vi "Log Current Register Values.vi"(7 "Unit ID (A)":string="A", 8 "error in":errorcluster, 10 "Use VI path? (T)":bool=TRUE, 11 "VISA Session In":refnum<visa-resource-name>="Alicat") -> (0 "error out":errorcluster, 3 "VISA Session Out":refnum<visa-resource-name>)   [LabVIEW 2014]
doc: "Reads off the value in each configuration/diagnostic register, and stores the values in a text file. Alicat saves a register log of each device before it leaves our facility; please contact us at (520) 290-6060 or by email at info@alicat.com if you are in need of this log file."
uses:
  <vilib>/Utility/file.llb/Write To Spreadsheet File (string).vi
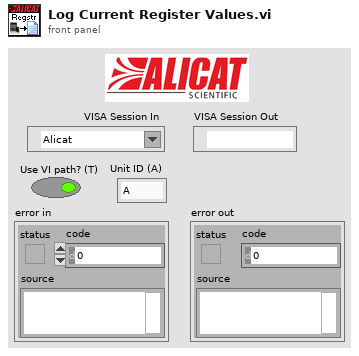
[diagram p1: front panel]
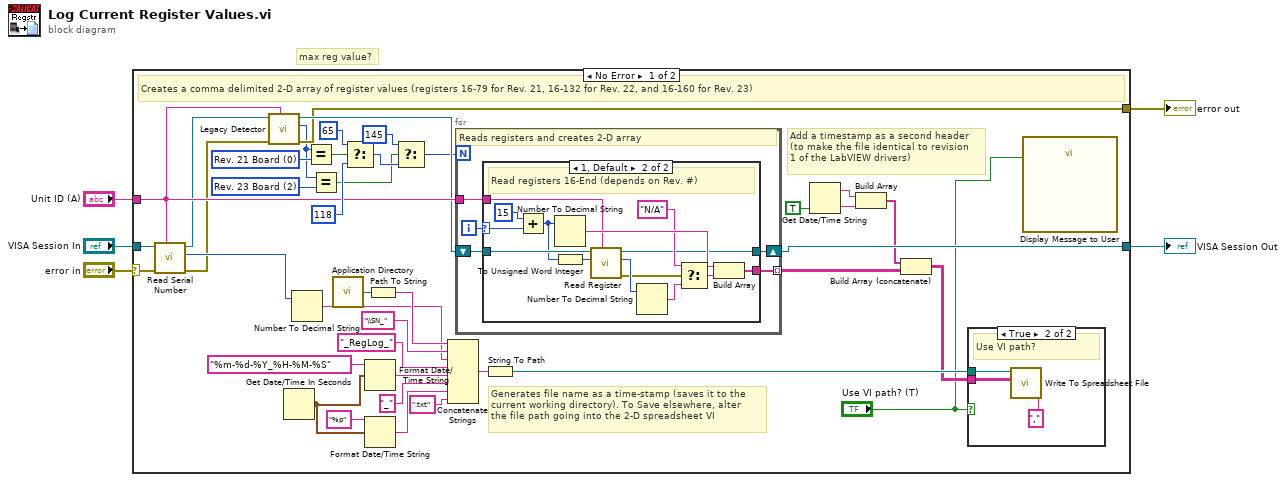
[diagram p0: block diagram]
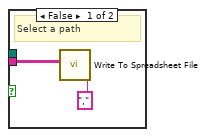
[diagram p2: hidden frame]
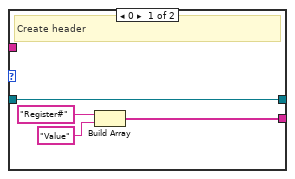
[diagram p3: hidden frame]
diagram:
  # "max reg value?"
  n1 = case shown="No Error" "error in" {
    selector: "error in" -> [w40 w75]
    tunnel: "VISA Session In" -> [w44 w74]
    tunnel: "Unit ID (A)" -> [w24 _]
    tunnel: [w43 w74] -> w3
    tunnel: [w20 w75] -> w2
    frame No Error {
      w9 = u8 2 items=["Rev. 21 Board", "Rev. 22 Board", "Rev. 23 Board"] ("Legacy Status")
      w45 = u8 0 items=["Rev. 21 Board", "Rev. 22 Board", "Rev. 23 Board"] ("Legacy Status")
      # "Add a timestamp as a second header\n(to make the file identical to revision\n1 of the LabVIEW drivers)"
      # "Generates file name as a time-stamp (saves it to the \ncurrent working directory). To Save elsewhere, alter\nthe file path going into the 2-D spreadsheet VI"
      # "Creates a comma delimited 2-D array of register values (registers 16-79 for Rev. 21, 16-132 for Rev. 22, and 16-160 for Rev. 23)"
      n2 = call "Read Serial Number.vi"("Unit ID (A)"=w24, "error in"=w40, "VISA Session In"=w44) -> ("error out"=w21:errorcluster, "Serial Number"=w26:i32, "VISA Session Out"=w23:refnum<visa-resource-name>)  [unwired: 6 in]
      n3 = call "Legacy Detector.vi"("Unit ID (A)"=w24, "error in"=w21, "VISA Session In"=w23) -> ("error out"=w20:errorcluster, "Legacy Status"=w8:u8, "VISA Session Out"=w22:refnum<visa-resource-name>)  [unwired: 6 in]
      n4 = Get Date/Time In Seconds() -> (seconds since 1Jan1904=w37:timestamp)
      n5 = Number To Decimal String(number=w26) -> (decimal integer string=w27:string)  [unwired: 1 in]
      n6 = Equal?(x=w8, y=w45) -> (x = y?=w10:bool)
      n7 = Equal?(x=w8, y=w9) -> (x = y?=w7:bool)
      n8 = call <vilib>:"Application Directory.vi"() -> ("Application Directory"=w31:path)
      n9 = Select(t=65, s=w10, f=118) -> (s? t:f=w12:i32)
      n10 = Format Date/Time String(time format string (%c)="%m-%d-%Y_%H-%M-%S", seconds (now)=w37) -> (date/time string=w36:string)  [unwired: 1 in]
      n11 = Format Date/Time String(time format string (%c)="%p", seconds (now)=w37) -> (date/time string=w35:string)  [unwired: 1 in]
      n12 = Path To String(path=w31) -> (string=w29:string)
      n13 = Select(t=145, s=w7, f=w12) -> (s? t:f=w11:i32)
      n14 = Concatenate Strings(w29, "\\SN_" ("string"), w27, "_RegLog_" ("string"), w36, "_" ("string"), w35, ".txt" ("string")) -> (w32:string)
      n15 = for {
        N: w11 -> [_]
        tunnel: [w52] -> w16 mode=indexing
        tunnel: w24 -> [w51]
        shift-right: [w53] -> w43
        shift-left: w22 -> [w54]
        i -> [w55]
        # "Reads registers and creates 2-D array"
        n16 = case shown="1, Default" w55 {
          selector: w55 -> [_ w73]
          tunnel: [w57 w70] -> w52
          tunnel: w54 -> [w56 w64]
          tunnel: [w56 w63] -> w53
          tunnel: w51 -> [_ w62]
          frame 0 {
            # "Create header"
            n17 = Build Array("Register#", "Value") -> (w57:string[])
          }
          frame 1, Default {
            # "Read registers 16-End (depends on Rev. #)"
            n18 = Add(x=15, y=w73) -> (x+y=w60:i32)
            n19 = Number To Decimal String(number=w60) -> (decimal integer string=w69:string)  [unwired: 1 in]
            n20 = To Unsigned Word Integer(number=w60) -> (unsigned 16bit integer=w61:u16)
            n21 = call "Read Register.vi"("Unit ID (A)"=w62, "Register address"=w61, "VISA Session In"=w64) -> ("error out"=w66:errorcluster, "Register Value (I32)"=w71:i32, "VISA Session Out"=w63:refnum<visa-resource-name>)  [unwired: 6 in]
            n22 = Number To Decimal String(number=w71) -> (decimal integer string=w67:string)  [unwired: 1 in]
            n23 = Select(t="N/A", s=w66, f=w67) -> (s? t:f=w68:string)
            n24 = Build Array(w69, w68) -> (w70:string[])
          }
        }
      }
      n25 = String To Path(string=w32) -> (path=w25:path)
      n26 = Get Date/Time String(want seconds? (F)=TRUE) -> (date string=w19:string, time string=w18:string)  [unwired: 2 in]
      n27 = Build Array(w19, w18) -> (w15:string[])
      n28 = Build Array (concatenate)(w15, w16) -> (w14:string[][])
      n29 = case shown="True" "Use VI path? (T)" {
        tunnel: w25 -> [_ w49]
        tunnel: w14 -> [w46 w48]
        frame False {
          # "Select a path"
          n30 = call-poly <vilib>:"Write To Spreadsheet File.vi"("delimiter (\\t)"="," ("delimiter (\\t)"), "2D data"=w46) -> ()  [unwired: 6 in, 1 out]
        }
        frame True {
          # "Use VI path?"
          n31 = call-poly <vilib>:"Write To Spreadsheet File.vi"("delimiter (\\t)"="," ("delimiter (\\t)"), "2D data"=w48, "file path (dialog if empty)"=w49) -> ()  [unwired: 5 in, 1 out]
        }
      }
      n32 = call "Display Message to User"("Enable"="Use VI path? (T)") -> ()  [unwired: 9 in, 2 out]
    }
    frame Error {
    }
  }
  "error out" <- w2
  "VISA Session Out" <- w3
